vi "KepcoDCPwr Interactive Example.vi"(11 "VISA resource name":refnum<visa-resource-name>="GPIB0::6::INSTR") -> ()   [LabVIEW 2013]
doc: "A complex example of the power supply operation showing all features of our products.\n\nSource code for function on buttons found in examples directory.\n\nversion 10.1"
uses:
  <vilib>/regexp/Match Regular Expression.xnode
panel:
  out "DC VOLTS 3":dbl=0.0258 format="%.3f"
  out "DC VOLTS 2":dbl=0.0258 format="%.3f"
  in  "Demo Mode Resistance - ( VISA resource name = BLANK )":dbl(slide) scale=0.0..10.0 scale format="%.1f"
  out "Instrument Error":errorcluster
  in  "Set Limits":bool
  out "Constant Voltage":bool=TRUE
  in  "Power Supply Mode":bool=TRUE
  in  "Arbitrary Waveform":bool
  in  "Function Generator":bool
  in  "Programmed List":bool
  in  "Software Ramp":bool
  in  "POWER":bool caption="STOP"
  in  "CURRENT":dbl(knob) min=-10.0 max=10.0 scale=-10.0..10.0 scale format="%.1f"
  out "DC AMPERES":dbl=-0.00061 format="%.3f"
  out "DC VOLTS":dbl=0.0258 format="%.3f"
  in  "DC\nOUTPUT":bool
  out "Output Enabled":bool
  in  "VOLTAGE":dbl(knob) min=-20.0 max=20.0 scale=-20.0..20.0 scale format="%.1f"
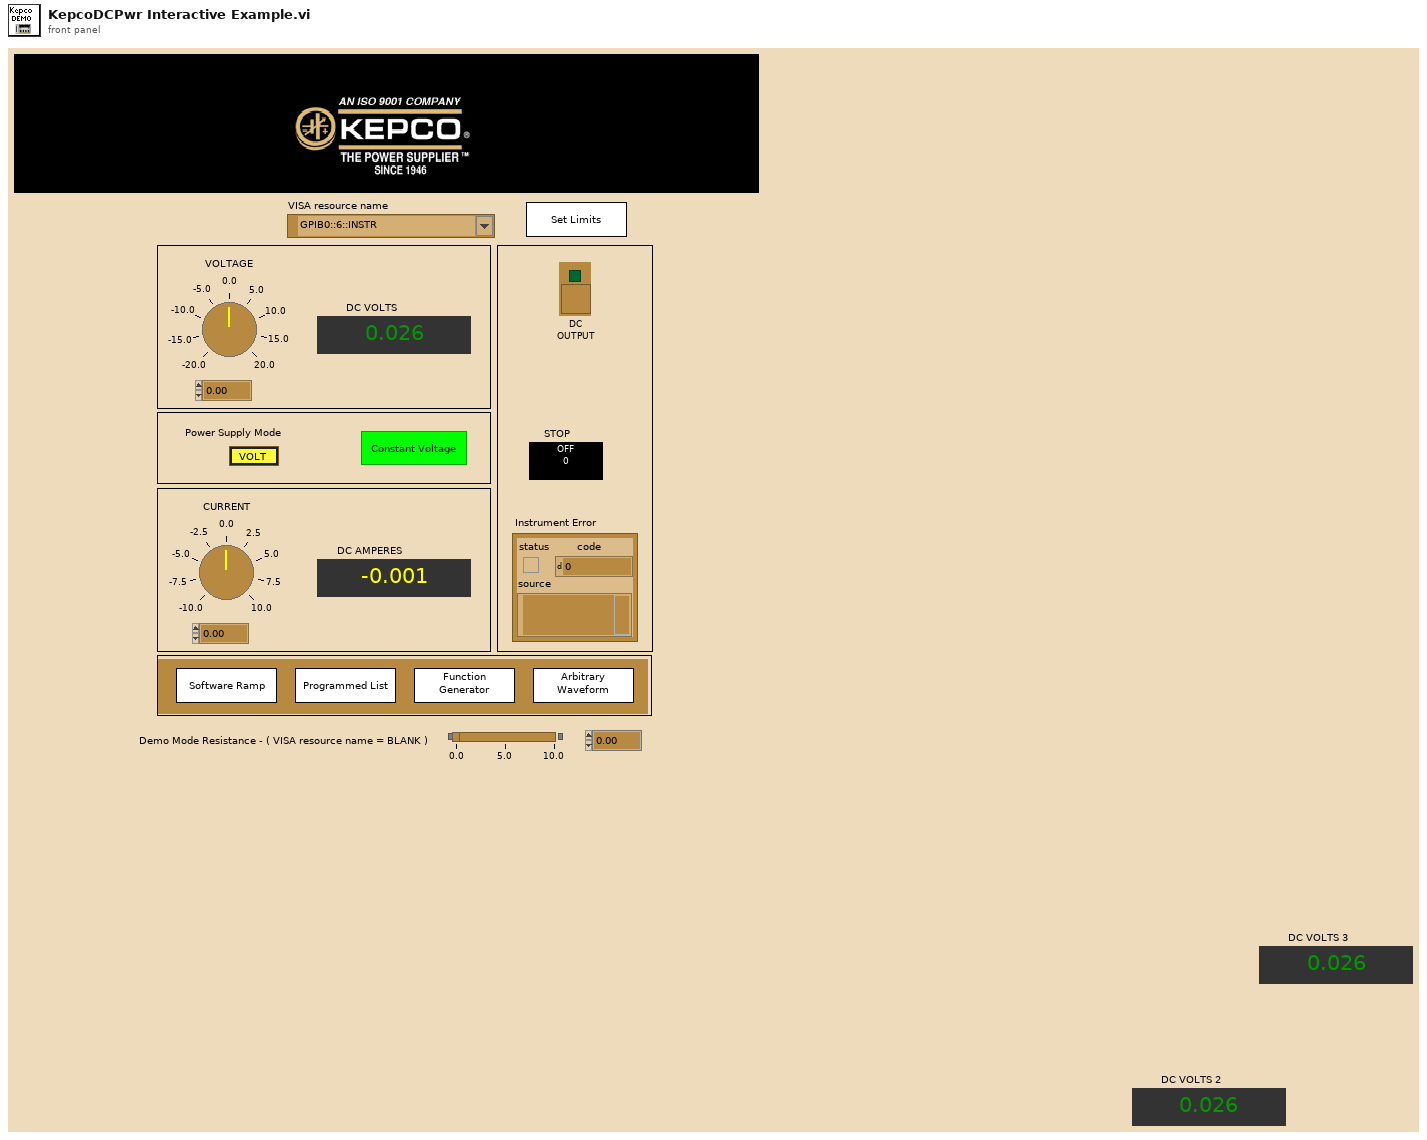
[diagram p1: front panel]
types:
  T1 = enum16{"Fixed", "List", "Transient", "External", "Gain", "Protect"}
  T2 = cluster{bool, "error code":i32, "error message":string}
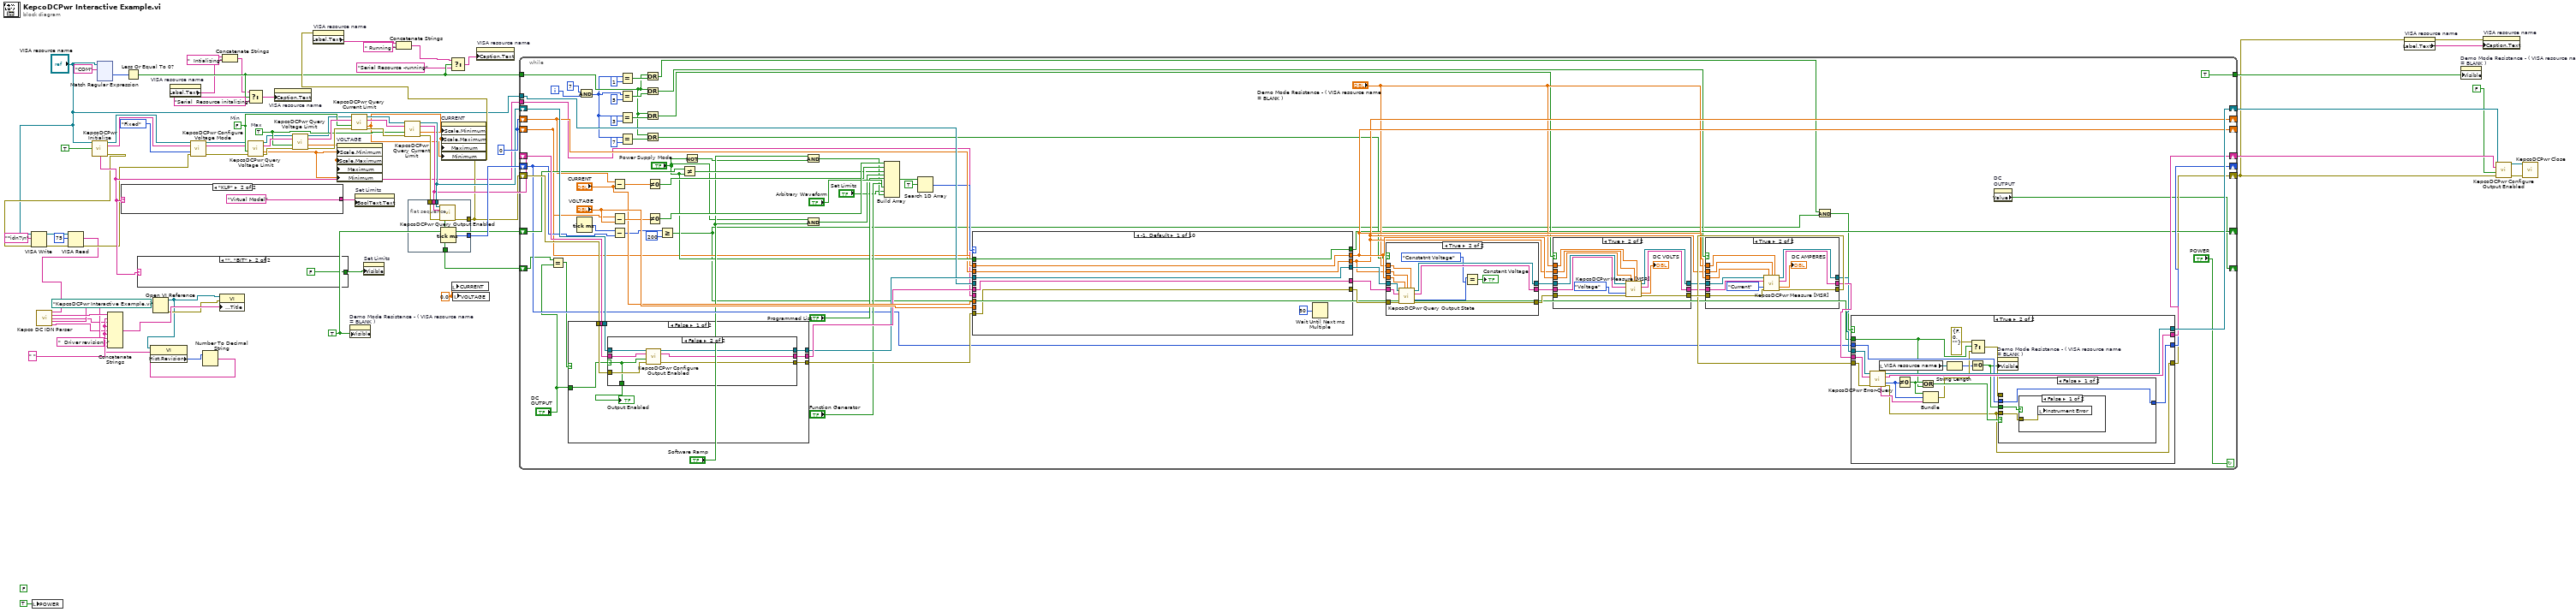
[diagram p0: block diagram]
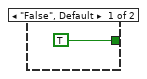
[diagram p2: hidden frame]
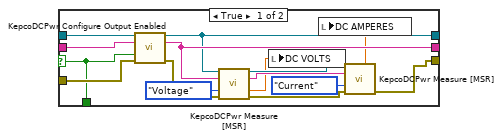
[diagram p3: hidden frame]
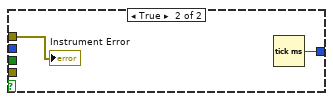
[diagram p7: hidden frame]
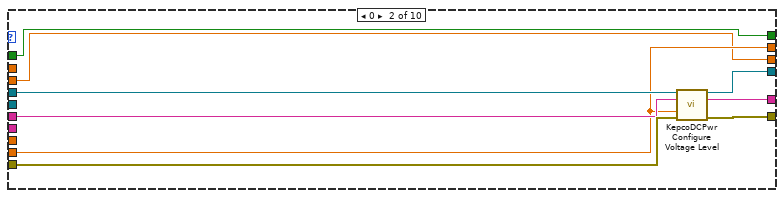
[diagram p11: hidden frame]
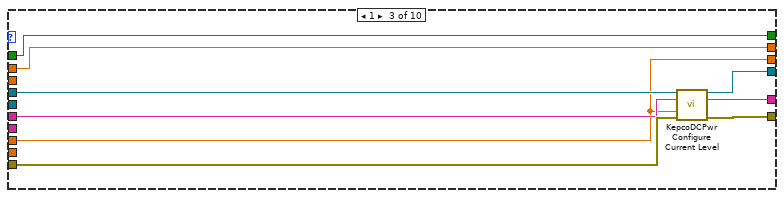
[diagram p12: hidden frame]
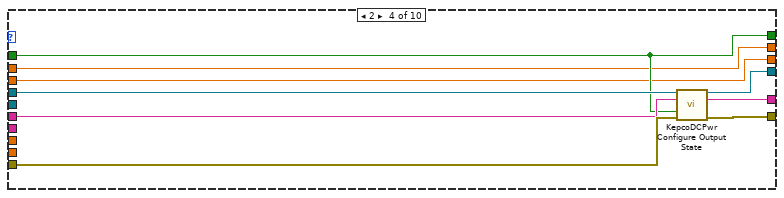
[diagram p13: hidden frame]
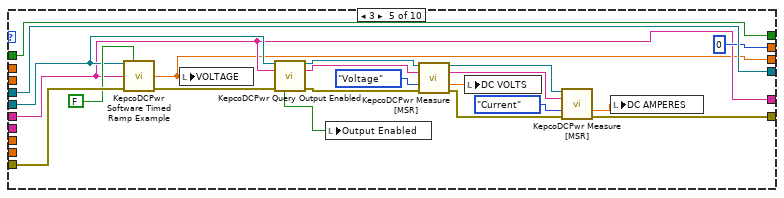
[diagram p14: hidden frame]
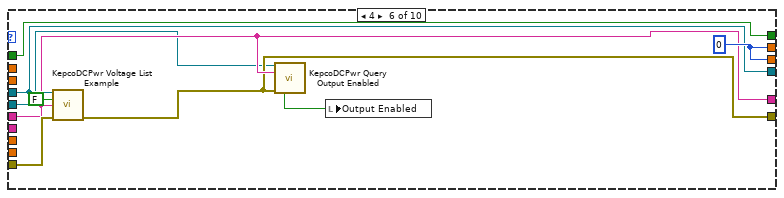
[diagram p15: hidden frame]
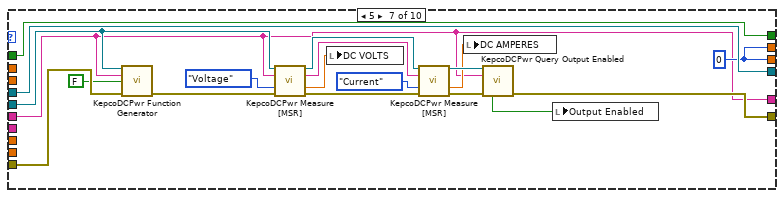
[diagram p16: hidden frame]
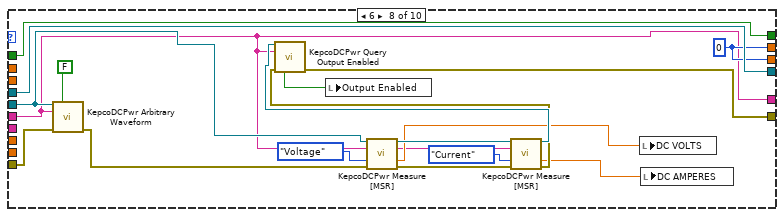
[diagram p17: hidden frame]
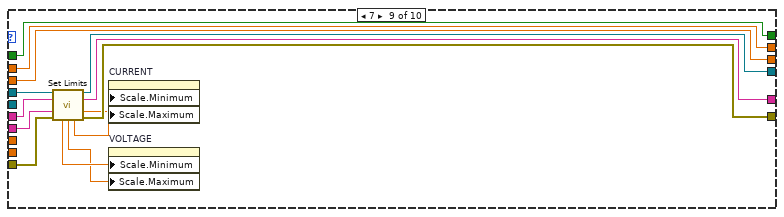
[diagram p18: hidden frame]
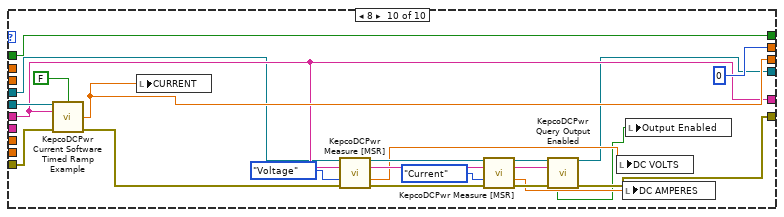
[diagram p19: hidden frame]
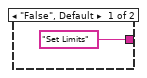
[diagram p20: hidden frame]
diagram:
  w11 = " " ("string")
  w31 = 0.0 ("VOLTAGE")
  (unwired) FALSE ("output enabled (True)")
  w58 = TRUE
  w60 = 0
  w69 = TRUE  # Max
  w70 = FALSE  # Min
  n1 = local write "POWER"(TRUE) -> ()
  n2 = call "KepcoDCPwr Initialize.vi"("VISA Resource Name"="VISA resource name", "id query (True)"=TRUE) -> ("VISA Session Out"=w57:refnum<visa-resource-name>, "Model Out"=w55:string, "Raw Model"=w26:string, "error out"=w22:errorcluster)  [unwired: 4 in, 6 out]
  n3 = VISA Write(VISA resource name="VISA resource name", write buffer="*idn?\n", error in (no error)=w22) -> (VISA resource name out=w24:refnum<visa-resource-name>, error out=w23:errorcluster)  [unwired: 1 out]
  n4 = VISA Read(VISA resource name=w24, byte count=u32 75, error in (no error)=w23) -> (read buffer=w19:string, error out=w20:errorcluster)  [unwired: 2 out]
  n5 = call "Kepco DC IDN Parser.vi"("IDN Query"=w19) -> ("Model"=w16:string, "Model #"=w9:string, "Firmware Version"=w12:string, "Serial Number"=w10:string)  [unwired: 9 in, 2 out]
  n6 = xnode "Match Regular Expression"("input string"="VISA resource name", "regular expression"="COM") -> ("offset past match"=w47:i32)  [unwired: 2 in, 6 out]
  n7 = case shown="\"KLP\"" w26 {
    tunnel: ["Set Limits" ("Boolean Text.Text") "Virtual Model" ("Boolean Text.Text")] -> w54
    frame "False", Default {
    }
    frame "KLP" {
    }
  }
  n8 = Less Or Equal To 0?(x=w47) -> (x <= 0?=w39:bool)
  n9 = case shown="\"\", \"BIT\"" w26 {
    tunnel: [TRUE ("Visible") FALSE ("Visible")] -> w25
    frame "False", Default {
    }
    frame "", "BIT" {
    }
  }
  n10 = Open VI Reference(vi path=path "KepcoDCPwr Interactive Example.vi") -> (vi reference=w7:refnum<vi>, error out=w13:errorcluster)  [unwired: 5 in]
  n11 = property class="VI"(reference=w7) -> ("Hist.Revision"=w6:u32)  [unwired: 1 in, 2 out]
  n12 = property on="VISA resource name" class="VISAName"() -> ("Label.Text"=w35:string)  [unwired: 2 in, 2 out]
  n13 = call "KepcoDCPwr Configure Voltage Mode.vi"("VISA Session"=w57, "Model In"=w55, "Mode (Fixed)"=T1."Fixed", "error in (no error)"=w20) -> ("VISA Session Out"=w63:refnum<visa-resource-name>, "Model Out"=w68:string, "error out"=w67:errorcluster)  [unwired: 2 in, 7 out]
  n14 = Number To Decimal String(number=w6) -> (decimal integer string=w5:string)  [unwired: 1 in]
  n15 = Concatenate Strings(w16, w11, w9, w11, w10, w11, w12, "  Driver revision  " ("string"), w5) -> (w15:string)
  n16 = property class="VI"(reference=w7, error in=w13, "Front Panel.Title"=w15) -> ()  [unwired: 2 out]
  n17 = Concatenate Strings(w35, "  Intializing" ("string")) -> (w34:string)
  n18 = Select(t=w34, s=w39, f="Serial  Resource initalizing") -> (s? t:f=w46:string)
  n19 = call "KepcoDCPwr Query Voltage Limit.vi"("VISA Session"=w63, "Model In"=w68, "Max Level (T),MIN LEVEL(F)"=w70, "error in (no error)"=w67) -> ("VISA Session Out"=w64:refnum<visa-resource-name>, "Model Out"=w75:string, "voltage level"=w30:dbl, "error out"=w76:errorcluster)  [unwired: 1 in, 7 out]
  n20 = property on="VISA resource name" class="VISAName"("Caption.Text"=w46) -> ()  [unwired: 2 in, 2 out]
  n21 = call "KepcoDCPwr Query Voltage Limit.vi"("VISA Session"=w64, "Model In"=w75, "Max Level (T),MIN LEVEL(F)"=w69, "error in (no error)"=w76) -> ("VISA Session Out"=w65:refnum<visa-resource-name>, "Model Out"=w71:string, "voltage level"=w29:dbl, "error out"=w74:errorcluster)  [unwired: 1 in, 7 out]
  n22 = property on="VISA resource name" class="VISAName"(error in=w40) -> ("Label.Text"=w4:string)  [unwired: 1 in, 2 out]
  n23 = property on="VOLTAGE" class="Knob (strict)"("Scale.Minimum"=w30, "Scale.Maximum"=w29, "Maximum"=w29, "Minimum"=w30) -> ()  [unwired: 2 in, 2 out]
  n24 = property on="Demo Mode Resistance - ( VISA resource name = BLANK )" class="Slide (strict)"("Visible"=w58) -> ()  [unwired: 2 in, 2 out]
  n25 = call "KepcoDCPwr Query Current Limit.vi"("VISA Session"=w65, "Model In"=w71, "Level"=w70, "error in (no error)"=w74) -> ("VISA Session Out"=w66:refnum<visa-resource-name>, "Model Out"=w72:string, "current limit"=w27:dbl, "error out"=w73:errorcluster)  [unwired: 1 in, 7 out]
  n26 = property on="Set Limits" class="Bool"("BoolText.Text"=w54) -> ()  [unwired: 2 in, 2 out]
  n27 = property on="Set Limits" class="Bool"("Visible"=w25) -> ()  [unwired: 2 in, 2 out]
  n28 = Concatenate Strings(w4, " Running " ("string")) -> (w32:string)
  n29 = call "KepcoDCPwr Query Current Limit.vi"("VISA Session"=w66, "Model In"=w72, "Level"=w69, "error in (no error)"=w73) -> ("VISA Session Out"=w44:refnum<visa-resource-name>, "Model Out"=w43:string, "current limit"=w28:dbl, "error out"=w42:errorcluster)  [unwired: 1 in, 7 out]
  n30 = flat-sequence {
    tunnel: [w87] -> w61
    tunnel: w44 -> [w86]
    tunnel: w43 -> [w85]
    tunnel: w42 -> [w84]
    tunnel: [w83] -> w41
    tunnel: [w82] -> w40
    frame #0 {
      n31 = call "KepcoDCPwr Query Output Enabled.vi"("VISA Session"=w86, "Model In"=w85, "error in (no error)"=w84) -> ("On"=w83:bool, "error out"=w82:errorcluster)  [unwired: 7 in, 4 out]
      n32 = Tick Count (ms)() -> (millisecond timer value=w87:u32)
    }
  }
  n33 = property on="CURRENT" class="Knob (strict)"("Scale.Minimum"=w27, "Scale.Maximum"=w28, "Maximum"=w28, "Minimum"=w27) -> ()  [unwired: 2 in, 2 out]
  n34 = Select(t=w32, s=w39, f="Serial Resource -running") -> (s? t:f=w38:string)
  n35 = local write "CURRENT"(w31) -> ()
  n36 = local write "VOLTAGE"(w31) -> ()
  n37 = property on="VISA resource name" class="VISAName"("Caption.Text"=w38) -> ()  [unwired: 2 in, 2 out]
  n38 = while {
    shift-left: w61 -> [w129]
    shift-right: [w130] -> _
    shift-left: w58 -> [w139]
    shift-right: [w125] -> _
    tunnel: "VISA resource name" -> [w149]
    shift-left: w60 -> [w117]
    shift-right: [w127] -> _
    shift-left: w60 -> [w118]
    shift-right: [w128] -> _
    shift-left: w43 -> [w155]
    shift-right: [w150] -> w50
    shift-left: w44 -> [w153]
    shift-right: [w151] -> w53
    shift-left: w40 -> [w157]
    shift-right: [w114] -> w2
    tunnel: [TRUE ("output enabled (True)")] -> w59
    tunnel: w26 -> [w110]
    tunnel: w39 -> [w96]
    shift-right: [w93] -> _
    shift-left: w41 -> [w94]
    i -> [w109]
    stop <- "POWER" continue-if-true
    n39 = Equal?(x=w94, y="DC\nOUTPUT") -> (x = y?=w91:bool)
    n40 = case shown="False" w91 {
      tunnel: w157 -> [w173 w198]
      tunnel: [w172 w198] -> w156
      tunnel: w155 -> [w171 w197]
      tunnel: [w170 w197] -> w154
      tunnel: w153 -> [w169 w196]
      tunnel: [w168 w196] -> w152
      tunnel: "DC\nOUTPUT" -> [w167 _]
      frame False {
        n41 = case shown="False" w167 {
          selector: w167 -> [w174 w189]
          tunnel: w173 -> [w188 w195]
          tunnel: [w179 w194] -> w172
          tunnel: w171 -> [w187 w193]
          tunnel: [w183 w192] -> w170
          tunnel: w169 -> [w186 w191]
          tunnel: [w182 w190] -> w168
          tunnel: [w174 w189] -> w166
          frame True {
            n42 = call "KepcoDCPwr Configure Output Enabled.vi"("VISA Session"=w186, "Model In"=w187, "Input enabled (True)"=w174, "error in (no error)"=w188) -> ("VISA Session Out"=w182:refnum<visa-resource-name>, "Model Out"=w183:string, "error out"=w181:errorcluster)  [unwired: 9 out]
            n43 = call "KepcoDCPwr Measure [MSR].vi"("VISA Session"=w182, "Model In"=w183, "measurement type (voltage)"=enum16{"Voltage", "Current"}."Voltage", "error in (no error)"=w181) -> ("VISA Session Out"=w185:refnum<visa-resource-name>, "Model Out"=w184:string, "measurement"=w178:dbl, "error out"=w180:errorcluster)  [unwired: 4 in, 4 out]
            n44 = local write "DC VOLTS"(w178) -> ()
            n45 = call "KepcoDCPwr Measure [MSR].vi"("VISA Session"=w185, "Model In"=w184, "measurement type (voltage)"=enum16{"Voltage", "Current"}."Current", "error in (no error)"=w180) -> ("measurement"=w175:dbl, "error out"=w179:errorcluster)  [unwired: 4 in, 6 out]
            n46 = local write "DC AMPERES"(w175) -> ()
          }
          frame False {
            n47 = call "KepcoDCPwr Configure Output Enabled.vi"("VISA Session"=w191, "Model In"=w193, "Input enabled (True)"=w189, "error in (no error)"=w195) -> ("VISA Session Out"=w190:refnum<visa-resource-name>, "Model Out"=w192:string, "error out"=w194:errorcluster)  [unwired: 9 out]
          }
        }
        "Output Enabled" <- w166
      }
      frame True {
      }
    }
    n48 = Tick Count (ms)() -> (millisecond timer value=w133:u32)
    n49 = And(x=7, y=w109) -> (x .and. y?=w95:i32)
    n50 = Subtract(x=w117, y="CURRENT") -> (x-y=w160:dbl)
    n51 = Subtract(x=w118, y="VOLTAGE") -> (x-y=w164:dbl)
    n52 = Subtract(x=w133, y=w129) -> (x-y=w132:u32)
    n53 = Equal?(x=w95, y=1) -> (x = y?=w97:bool)
    n54 = Equal?(x=w95, y=5) -> (x = y?=w101:bool)
    n55 = Equal?(x=w95, y=3) -> (x = y?=w103:bool)
    n56 = Equal?(x=w95, y=7) -> (x = y?=w106:bool)
    n57 = Or(x=w96, y=w97) -> (x .or. y?=w89:bool)
    n58 = Or(x=w96, y=w101) -> (x .or. y?=w99:bool)
    n59 = Or(x=w96, y=w103) -> (x .or. y?=w102:bool)
    n60 = Or(x=w96, y=w106) -> (x .or. y?=w105:bool)
    n61 = Not Equal To 0?(x=w160) -> (x != 0?=w158:bool)
    n62 = Not Equal To 0?(x=w164) -> (x != 0?=w163:bool)
    n63 = Greater Or Equal?(x=w132, y=u32 200) -> (x >= y?=w90:bool)
    n64 = Not Equal?(x=w139, y="Power Supply Mode") -> (x != y?=w138:bool)
    n65 = Not(x="Power Supply Mode") -> (.not. x?=w121:bool)
    n66 = And(x="Software Ramp", y=w121) -> (x .and. y?=w123:bool)
    n67 = And(x="Power Supply Mode", y="Software Ramp") -> (x .and. y?=w124:bool)
    n68 = Build Array(w163, w158, w138, w124, "Programmed List", "Function Generator", "Arbitrary Waveform", "Set Limits", w123) -> (w162:bool[])
    n69 = Search 1D Array(1D array=w162, element=TRUE) -> (index of element=w112:i32)  [unwired: 1 in]
    n70 = case shown="-1, Default" w112 {
      tunnel: "VOLTAGE" -> [_ w280 _ _ _ _ _ _ _ _]
      tunnel: [w272 w280 w287 w297 0 w333 w350 w369 w375 0] -> w128
      tunnel: w152 -> [w277 w284 w293 w302 w325 w332 w353 w372 w383 w390]
      tunnel: w154 -> [w276 w285 w294 w303 w319 w328 w335 w354 w381 w396]
      tunnel: w156 -> [w275 w286 w295 w304 w324 w331 w352 w371 w385 w408]
      tunnel: [w277 w283 w292 w301 w325 w332 w353 w372 w382 w389] -> w136
      tunnel: [w276 w282 w291 w300 w319 w328 w335 w354 w380 w396] -> w135
      tunnel: [w275 w281 w290 w299 w310 w327 w348 w367 w384 w388] -> w116
      tunnel: "CURRENT" -> [_ _ w289 _ _ _ _ _ _ _]
      tunnel: [w271 w278 w289 w296 w305 w333 w350 w369 w374 w403] -> w127
      tunnel: w149 -> [_ _ _ _ w320 w326 w338 w363 _ w407]
      tunnel: "Power Supply Mode" -> [w273 w279 w288 w298 w323 w334 w351 w370 w386 w406]
      tunnel: [w273 w279 w288 w298 w323 w334 w351 w370 w386 w406] -> w125
      tunnel: w118 -> [w272 _ w287 w297 _ _ _ _ w375 _]
      tunnel: w117 -> [w271 w278 _ w296 _ _ _ _ w374 _]
      tunnel: w110 -> [_ _ _ _ _ _ _ _ w373 _]
      frame -1, Default {
        n71 = Wait Until Next ms Multiple(millisecond multiple=u32 50 ("milliseconds to wait")) -> ()  [unwired: 1 out]
      }
      frame 0 {
        n72 = call "KepcoDCPwr Configure Voltage Level.vi"("VISA Session"=w284, "Model In"=w285, "level (0.0 volts)"=w280, "error in (no error)"=w286) -> ("VISA Session Out"=w283:refnum<visa-resource-name>, "Model Out"=w282:string, "error out"=w281:errorcluster)  [unwired: 1 in, 8 out]
      }
      frame 1 {
        n73 = call "KepcoDCPwr Configure Current Level.vi"("VISA Session"=w293, "Model In"=w294, "level (0.0 volts)"=w289, "error in (no error)"=w295) -> ("VISA Session Out"=w292:refnum<visa-resource-name>, "Model Out"=w291:string, "error out"=w290:errorcluster)  [unwired: 1 in, 8 out]
      }
      frame 2 {
        n74 = call "KepcoDCPwr Configure Output State.vi"("VISA Session"=w302, "Model In"=w303, "Power Supply Mode"=w298, "error in (no error)"=w304) -> ("VISA Session Out"=w301:refnum<visa-resource-name>, "Model Out"=w300:string, "error out"=w299:errorcluster)  [unwired: 1 in, 8 out]
      }
      frame 3 {
        n75 = call "KepcoDCPwr Software Timed Ramp Example.vi"("VISA resource name"=w320, "Boolean"=FALSE, "Model In"=w319, "error in (no error)"=w324) -> ("End voltage"=w305:dbl, "error out"=w318:errorcluster)  [unwired: 10 out]
        n76 = local write "VOLTAGE"(w305) -> ()
        n77 = call "KepcoDCPwr Query Output Enabled.vi"("VISA Session"=w320, "Model In"=w319, "error in (no error)"=w318) -> ("VISA Session Out"=w314:refnum<visa-resource-name>, "Model Out"=w315:string, "On"=w317:bool, "error out"=w316:errorcluster)  [unwired: 7 in, 2 out]
        n78 = local write "Output Enabled"(w317) -> ()
        n79 = call "KepcoDCPwr Measure [MSR].vi"("VISA Session"=w314, "Model In"=w315, "measurement type (voltage)"=enum16{"Voltage", "Current"}."Voltage", "error in (no error)"=w316) -> ("VISA Session Out"=w312:refnum<visa-resource-name>, "Model Out"=w313:string, "measurement"=w309:dbl, "error out"=w311:errorcluster)  [unwired: 4 in, 4 out]
        n80 = local write "DC VOLTS"(w309) -> ()
        n81 = call "KepcoDCPwr Measure [MSR].vi"("VISA Session"=w312, "Model In"=w313, "measurement type (voltage)"=enum16{"Voltage", "Current"}."Current", "error in (no error)"=w311) -> ("measurement"=w308:dbl, "error out"=w310:errorcluster)  [unwired: 4 in, 6 out]
        n82 = local write "DC AMPERES"(w308) -> ()
      }
      frame 4 {
        w333 = 0
        n83 = call "KepcoDCPwr Voltage List Example.vi"("VISA resource name"=w332, "Open & close"=FALSE, "Model In"=w328, "error in (no error)"=w331) -> ("error out"=w327:errorcluster)  [unwired: 11 in]
        n84 = call "KepcoDCPwr Query Output Enabled.vi"("VISA Session"=w326, "Model In"=w328, "error in (no error)"=w327) -> ("On"=w330:bool)  [unwired: 7 in, 5 out]
        n85 = local write "Output Enabled"(w330) -> ()
      }
      frame 5 {
        w350 = 0
        n86 = call "KepcoDCPwr Function Generator.vi"("VISA resource name"=w338, "Model Out"=w335, "Standalone"=FALSE, "error in (no error)"=w352) -> ("error out"=w339:errorcluster)  [unwired: 11 out]
        n87 = call "KepcoDCPwr Measure [MSR].vi"("VISA Session"=w338, "Model In"=w335, "measurement type (voltage)"=enum16{"Voltage", "Current"}."Voltage", "error in (no error)"=w339) -> ("VISA Session Out"=w346:refnum<visa-resource-name>, "Model Out"=w345:string, "measurement"=w336:dbl, "error out"=w344:errorcluster)  [unwired: 4 in, 4 out]
        n88 = local write "DC VOLTS"(w336) -> ()
        n89 = call "KepcoDCPwr Measure [MSR].vi"("VISA Session"=w346, "Model In"=w345, "measurement type (voltage)"=enum16{"Voltage", "Current"}."Current", "error in (no error)"=w344) -> ("VISA Session Out"=w343:refnum<visa-resource-name>, "measurement"=w337:dbl, "error out"=w342:errorcluster)  [unwired: 4 in, 5 out]
        n90 = local write "DC AMPERES"(w337) -> ()
        n91 = call "KepcoDCPwr Query Output Enabled.vi"("VISA Session"=w343, "Model In"=w335, "error in (no error)"=w342) -> ("On"=w349:bool, "error out"=w348:errorcluster)  [unwired: 7 in, 4 out]
        n92 = local write "Output Enabled"(w349) -> ()
      }
      frame 6 {
        w369 = 0
        n93 = call "KepcoDCPwr Arbitrary Waveform.vi"("VISA resource name"=w363, "Open / Close"=FALSE, "Model In"=w354, "error in (no error)"=w371) -> ("error out"=w360:errorcluster)  [unwired: 11 in]
        n94 = call "KepcoDCPwr Measure [MSR].vi"("VISA Session"=w363, "Model In"=w354, "measurement type (voltage)"=enum16{"Voltage", "Current"}."Voltage", "error in (no error)"=w360) -> ("VISA Session Out"=w362:refnum<visa-resource-name>, "Model Out"=w355:string, "measurement"=w357:dbl, "error out"=w366:errorcluster)  [unwired: 4 in, 4 out]
        n95 = call "KepcoDCPwr Measure [MSR].vi"("VISA Session"=w362, "Model In"=w355, "measurement type (voltage)"=enum16{"Voltage", "Current"}."Current", "error in (no error)"=w366) -> ("VISA Session Out"=w361:refnum<visa-resource-name>, "measurement"=w358:dbl, "error out"=w359:errorcluster)  [unwired: 4 in, 5 out]
        n96 = call "KepcoDCPwr Query Output Enabled.vi"("VISA Session"=w361, "Model In"=w354, "error in (no error)"=w359) -> ("On"=w368:bool, "error out"=w367:errorcluster)  [unwired: 7 in, 4 out]
        n97 = local write "Output Enabled"(w368) -> ()
        n98 = local write "DC VOLTS"(w357) -> ()
        n99 = local write "DC AMPERES"(w358) -> ()
      }
      frame 7 {
        n100 = call "Set Limits.vi"("VISA Session"=w383, "Model In"=w381, "Raw Model In"=w373, "error in (no error)"=w385) -> ("VISA Session Out"=w382:refnum<visa-resource-name>, "Model Out"=w380:string, "Max Current Limit"=w376:dbl, "Min Voltage Limit"=w379:dbl, "Max Voltage Limit"=w378:dbl, "Min Current Limit"=w377:dbl, "error out"=w384:errorcluster)  [unwired: 1 in, 4 out]
        n101 = property on="CURRENT" class="Knob (strict)"("Scale.Minimum"=w377, "Scale.Maximum"=w376) -> ()  [unwired: 2 in, 2 out]
        n102 = property on="VOLTAGE" class="Knob (strict)"("Scale.Minimum"=w379, "Scale.Maximum"=w378) -> ()  [unwired: 2 in, 2 out]
      }
      frame 8 {
        n103 = call "KepcoDCPwr Current Software Timed Ramp Example.vi"("VISA resource name"=w407, "OPpen/Close"=FALSE, "Model In"=w396, "error in (no error)"=w408) -> ("actual current"=w403:dbl, "error out"=w397:errorcluster)  [unwired: 10 out]
        n104 = local write "CURRENT"(w403) -> ()
        n105 = call "KepcoDCPwr Measure [MSR].vi"("VISA Session"=w390, "Model In"=w396, "measurement type (voltage)"=enum16{"Voltage", "Current"}."Voltage", "error in (no error)"=w397) -> ("VISA Session Out"=w394:refnum<visa-resource-name>, "Model Out"=w395:string, "measurement"=w392:dbl, "error out"=w398:errorcluster)  [unwired: 4 in, 4 out]
        n106 = call "KepcoDCPwr Measure [MSR].vi"("VISA Session"=w394, "Model In"=w395, "measurement type (voltage)"=enum16{"Voltage", "Current"}."Current", "error in (no error)"=w398) -> ("VISA Session Out"=w399:refnum<visa-resource-name>, "Model Out"=w393:string, "measurement"=w391:dbl, "error out"=w400:errorcluster)  [unwired: 4 in, 4 out]
        n107 = call "KepcoDCPwr Query Output Enabled.vi"("VISA Session"=w399, "Model In"=w393, "error in (no error)"=w400) -> ("VISA Session Out"=w389:refnum<visa-resource-name>, "On"=w387:bool, "error out"=w388:errorcluster)  [unwired: 7 in, 3 out]
        n108 = local write "DC VOLTS"(w392) -> ()
        n109 = local write "DC AMPERES"(w391) -> ()
        n110 = local write "Output Enabled"(w387) -> ()
      }
    }
    n111 = case shown="True" w105 {
      tunnel: [w258 w270] -> w137
      tunnel: w136 -> [w258 w269]
      tunnel: w135 -> [w257 w268]
      tunnel: [w257 w267] -> w134
      tunnel: w128 -> [_ w264]
      tunnel: w127 -> [_ w263]
      tunnel: "Demo Mode Resistance - ( VISA resource name = BLANK )" -> [_ w262]
      tunnel: w116 -> [w256 w261]
      tunnel: [w256 w260] -> w115
      frame False {
      }
      frame True {
        n112 = call "KepcoDCPwr Query Output State.vi"("VISA Session"=w269, "Virtual Voltage"=w264, "Virtual Current"=w263, "Virtual Resistance"=w262, "Model In"=w268, "error in (no error)"=w261) -> ("VISA Session Out"=w270:refnum<visa-resource-name>, "Model Out"=w267:string, "Output state (Constant Voltage)"=w265:enum16{"Constatnt Voltage", "Constant Current"}, "error out"=w260:errorcluster)  [unwired: 2 in, 4 out]
        n113 = Equal?(x=w265, y=enum16{"Constatnt Voltage", "Constant Current"}."Constatnt Voltage" ("Output state (Constant Voltage)")) -> (x = y?=→"Constant Voltage":bool)
      }
    }
    n114 = case shown="True" w102 {
      tunnel: [w242 w253] -> w148
      tunnel: [w243 w252] -> w145
      tunnel: [w244 w251] -> w143
      tunnel: w137 -> [w244 w250]
      tunnel: w134 -> [w243 w249]
      tunnel: w128 -> [_ w248]
      tunnel: w127 -> [_ w247]
      tunnel: "Demo Mode Resistance - ( VISA resource name = BLANK )" -> [_ w246]
      tunnel: w115 -> [w242 w245]
      frame False {
      }
      frame True {
        n115 = call "KepcoDCPwr Measure [MSR].vi"("VISA Session"=w250, "Virtual Voltage"=w248, "Virtual Current"=w247, "Virtual Resistance"=w246, "Model In"=w249, "measurement type (voltage)"=enum16{"Voltage", "Current"}."Voltage", "error in (no error)"=w245) -> ("VISA Session Out"=w251:refnum<visa-resource-name>, "Model Out"=w252:string, "measurement"=→"DC VOLTS":dbl, "error out"=w253:errorcluster)  [unwired: 1 in, 4 out]
      }
    }
    n116 = case shown="True" w99 {
      tunnel: w148 -> [w228 w239]
      tunnel: [w228 w238] -> w147
      tunnel: [w229 w237] -> w146
      tunnel: w145 -> [w229 w236]
      tunnel: [w230 w235] -> w144
      tunnel: w143 -> [w230 w234]
      tunnel: w128 -> [_ w233]
      tunnel: w127 -> [_ w232]
      tunnel: "Demo Mode Resistance - ( VISA resource name = BLANK )" -> [_ w231]
      frame False {
      }
      frame True {
        n117 = call "KepcoDCPwr Measure [MSR].vi"("VISA Session"=w234, "Virtual Voltage"=w233, "Virtual Current"=w232, "Virtual Resistance"=w231, "Model In"=w236, "measurement type (voltage)"=enum16{"Voltage", "Current"}."Current", "error in (no error)"=w239) -> ("VISA Session Out"=w235:refnum<visa-resource-name>, "Model Out"=w237:string, "measurement"=→"DC AMPERES":dbl, "error out"=w238:errorcluster)  [unwired: 1 in, 4 out]
      }
    }
    n118 = And(x=w89, y=w90) -> (x .and. y?=w88:bool)
    n119 = case shown="True" w88 {
      tunnel: [w201 w221] -> w151
      tunnel: [w200 w220] -> w150
      tunnel: w147 -> [w202 w219]
      tunnel: w146 -> [w200 w218]
      tunnel: w144 -> [w201 w217]
      tunnel: [w199 w216] -> w130
      tunnel: w129 -> [w199 w215]
      tunnel: w90 -> [_ w210]
      tunnel: [w202 w206] -> w114
      frame False {
      }
      frame True {
        n120 = call "KepcoDCPwr Error-Query.vi"("VISA Session"=w217, "Model In"=w218, "error in (no error)"=w219) -> ("VISA Session Out"=w221:refnum<visa-resource-name>, "Model Out"=w220:string, "error code"=w212:i32, "error message"=w213:string, "error out"=w206:errorcluster)  [unwired: 1 in, 7 out]
        n121 = local read "VISA resource name"() -> (w205:refnum<visa-resource-name>)
        n122 = Not Equal To 0?(x=w212) -> (x != 0?=w211:bool)
        n123 = Or(x=w211, y=w210) -> (x .or. y?=w214:bool)
        n124 = Bundle(w211, "error code"=w212, "error message"=w213) -> (w209:T2)  [unwired: 1 out]
        n125 = String Length(string=w205) -> (length=w204:i32)
        n126 = Select(t=T2 {FALSE, "error code"=0, "error message"=""}, s=w210, f=w209) -> (s? t:f=w208:T2)
        n127 = Equal To 0?(x=w204) -> (x = 0?=w203:bool)
        n128 = property on="Demo Mode Resistance - ( VISA resource name = BLANK )" class="Slide (strict)"("Visible"=w203) -> ()  [unwired: 2 in, 2 out]
        n129 = case shown="False" w214 {
          tunnel: [w224 w227] -> w216
          tunnel: w215 -> [w224 _]
          tunnel: w208 -> [_ w226]
          tunnel: w206 -> [w223 _]
          tunnel: w203 -> [w222 _]
          frame False {
            n130 = case shown="False" w222 {
              tunnel: w223 -> [w225 _]
              frame False {
                n131 = local write "Instrument Error"(w225) -> ()
              }
              frame True {
              }
            }
          }
          frame True {
            n132 = Tick Count (ms)() -> (millisecond timer value=w227:u32)
            "Instrument Error" <- w226
          }
        }
      }
    }
    n133 = property on="DC\nOUTPUT" class="Bool (strict)"() -> ("Value"=w93:bool)  [unwired: 2 in, 2 out]
  }
  n134 = property on="VISA resource name" class="VISAName"(error in=w2) -> (error out=w1:errorcluster, "Label.Text"=w3:string)  [unwired: 1 in, 1 out]
  n135 = property on="Demo Mode Resistance - ( VISA resource name = BLANK )" class="Slide (strict)"("Visible"=w59) -> ()  [unwired: 2 in, 2 out]
  n136 = property on="VISA resource name" class="VISAName"(error in=w1, "Caption.Text"=w3) -> ()  [unwired: 1 in, 2 out]
  n137 = call "KepcoDCPwr Configure Output Enabled.vi"("VISA Session"=w53, "Model In"=w50, "Input enabled (True)"=FALSE, "error in (no error)"=w2) -> ("VISA Session Out"=w51:refnum<visa-resource-name>, "error out"=w52:errorcluster)  [unwired: 10 out]
  n138 = call "KepcoDCPwr Close.vi"("VISA Session"=w51, "error in (no error)"=w52) -> ()  [unwired: 14 out]
